vi "MainPanel_20170525.vi"() -> (0 "ErrorOut":errorcluster)   [LabVIEW 2018] (continued)
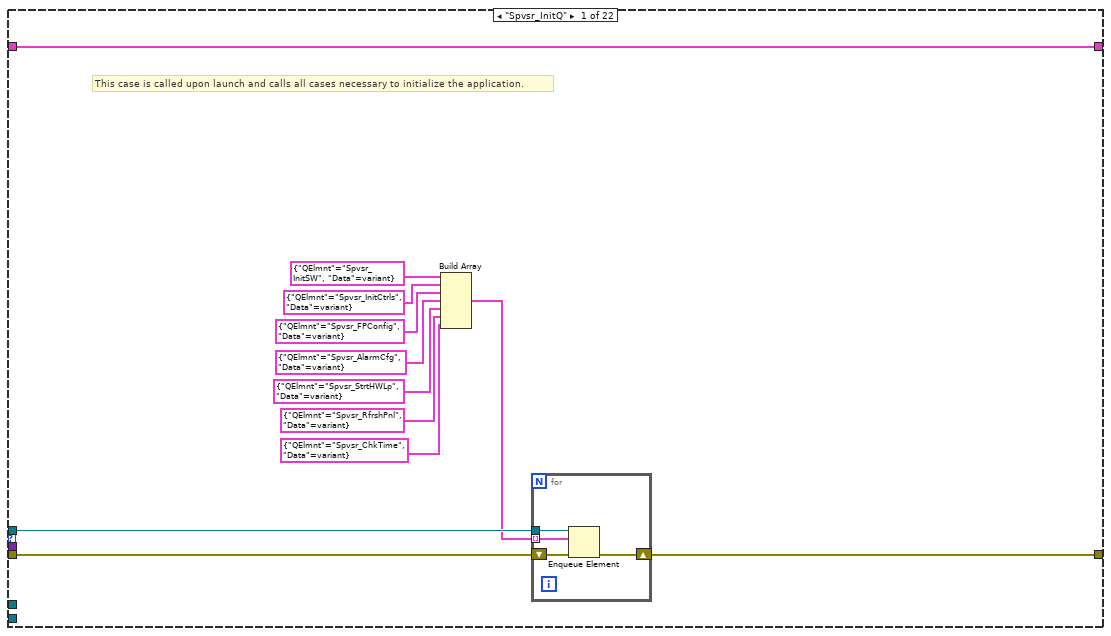
[diagram p3: hidden frame]
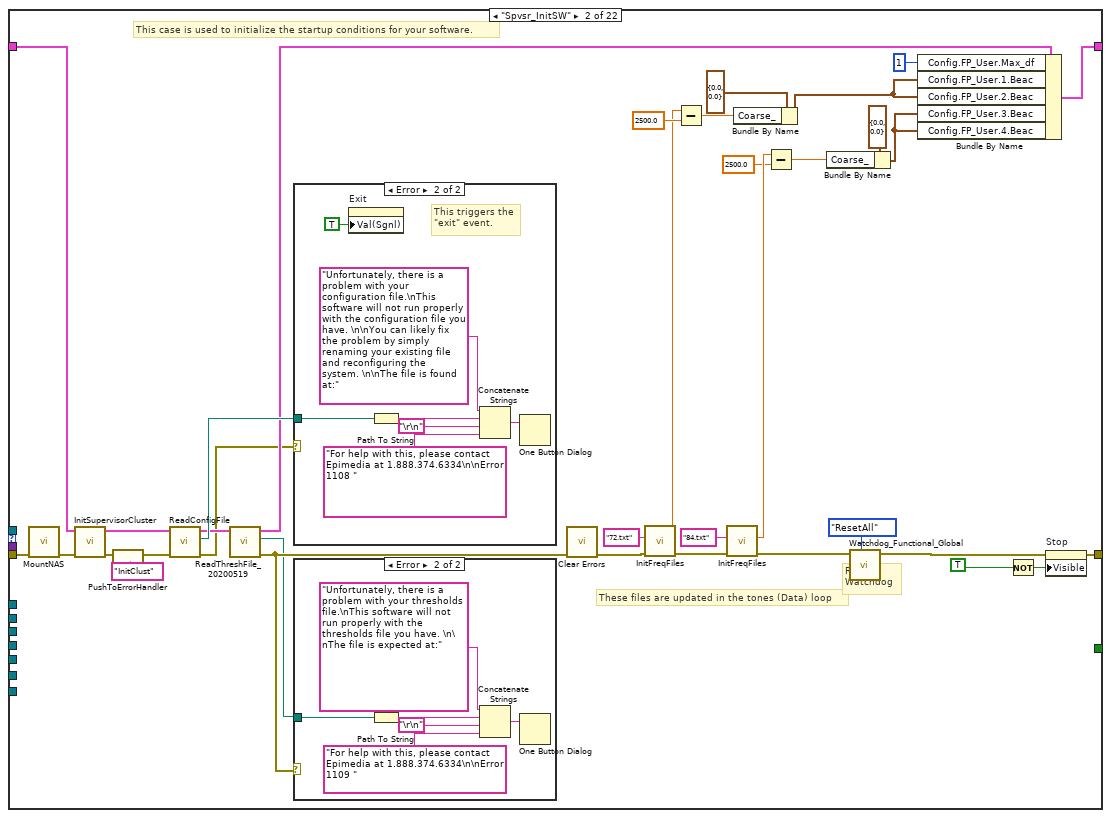
[diagram p4: hidden frame]
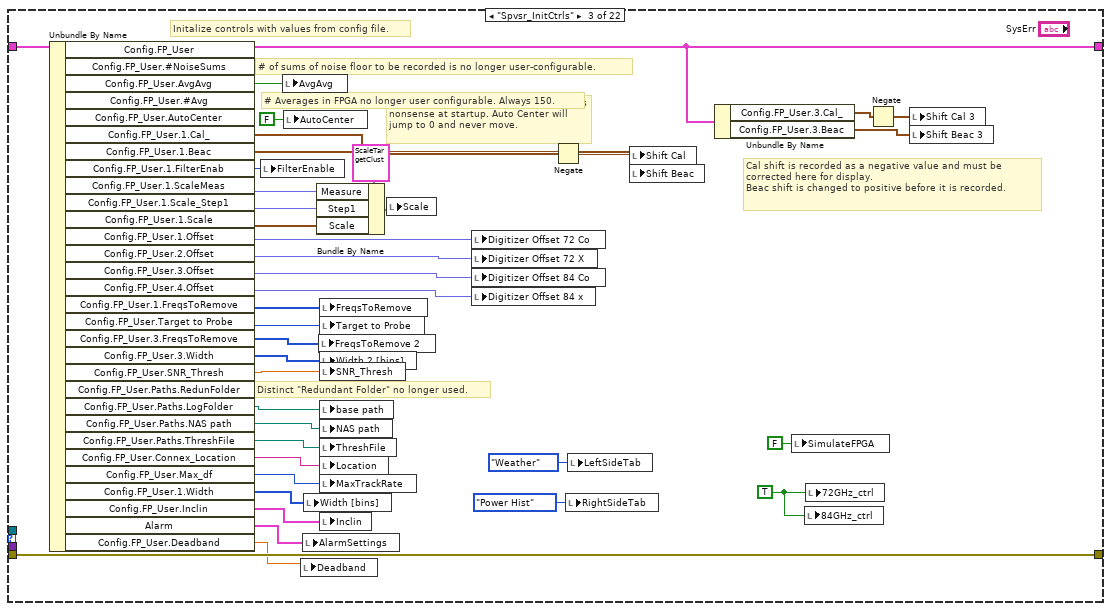
[diagram p7: hidden frame]
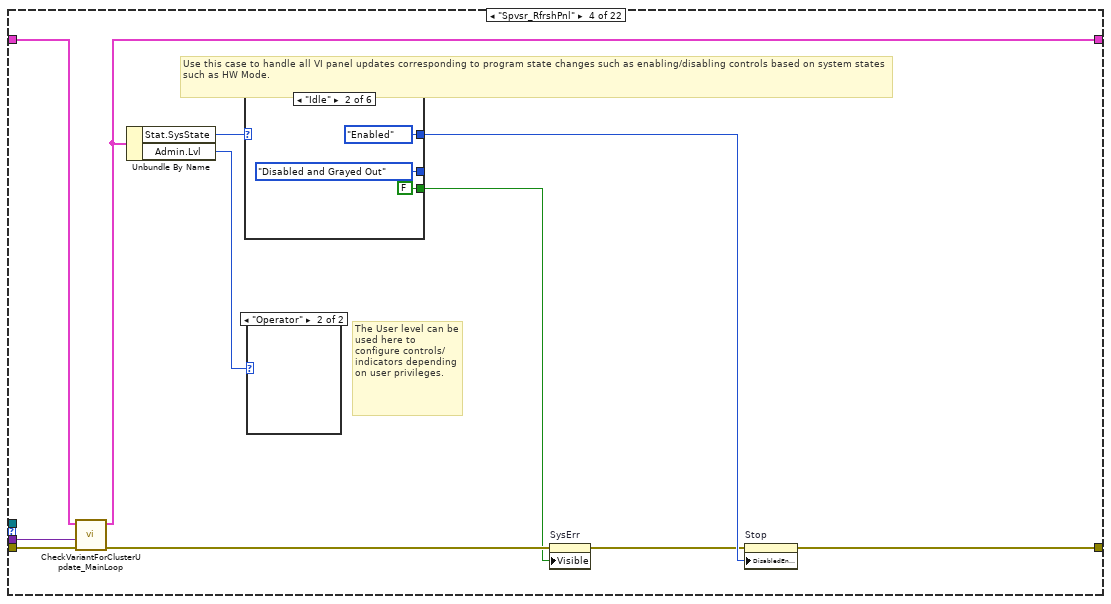
[diagram p8: hidden frame]
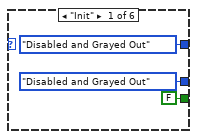
[diagram p10: hidden frame]
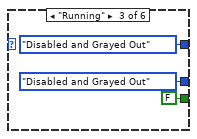
[diagram p11: hidden frame]
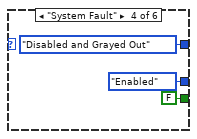
[diagram p12: hidden frame]
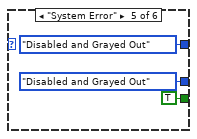
[diagram p13: hidden frame]
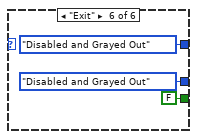
[diagram p14: hidden frame]
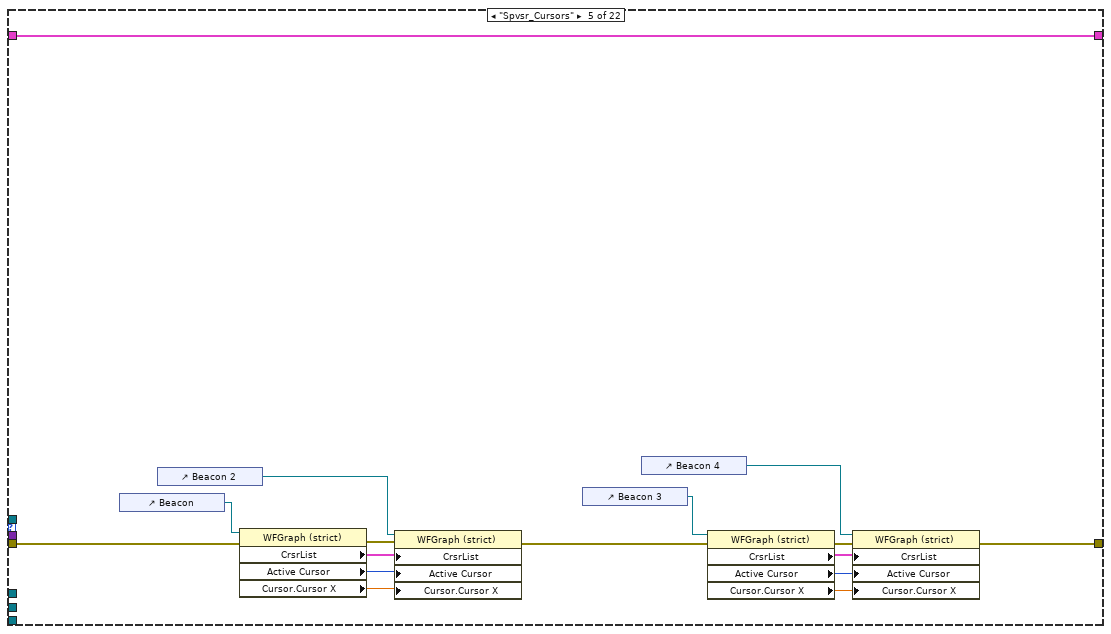
[diagram p15: hidden frame]
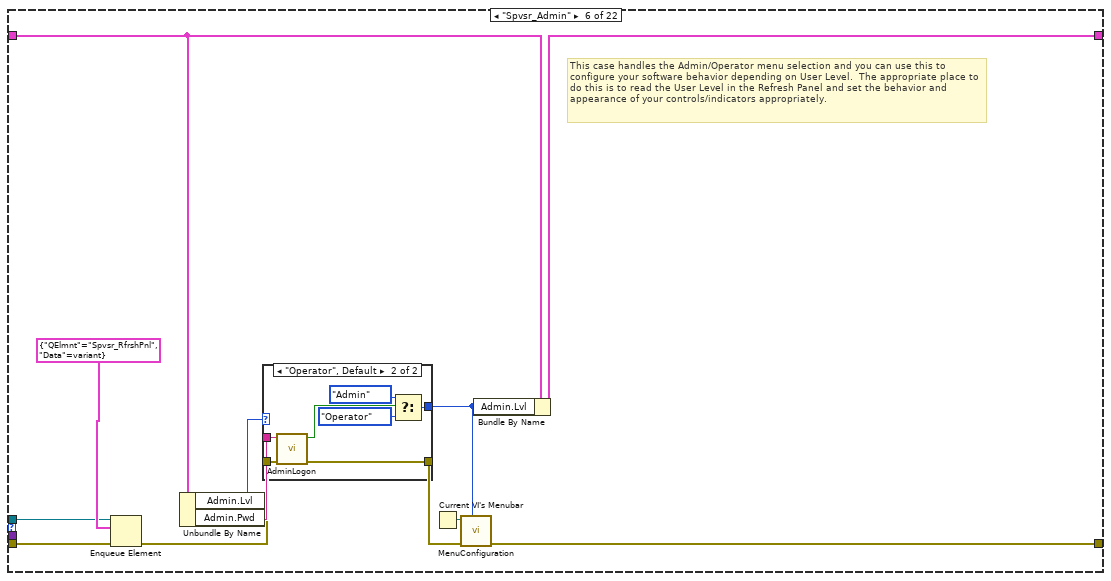
[diagram p16: hidden frame]
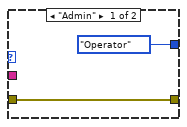
[diagram p17: hidden frame]
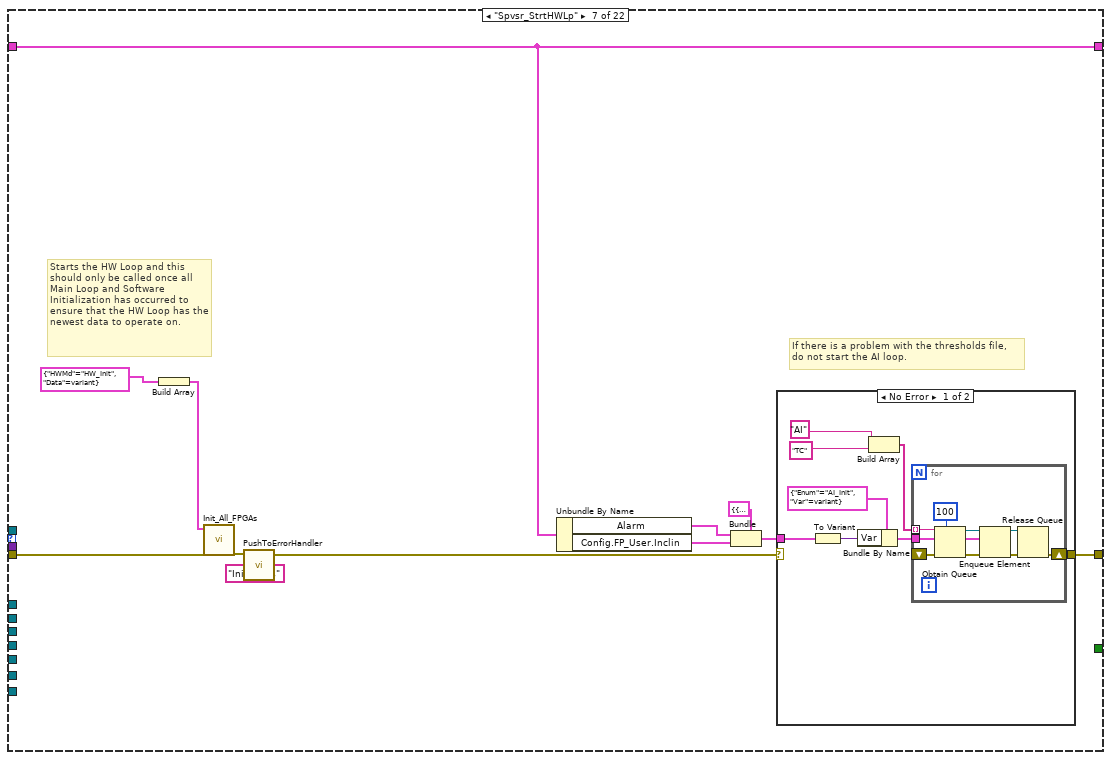
[diagram p18: hidden frame]
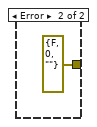
[diagram p19: hidden frame]
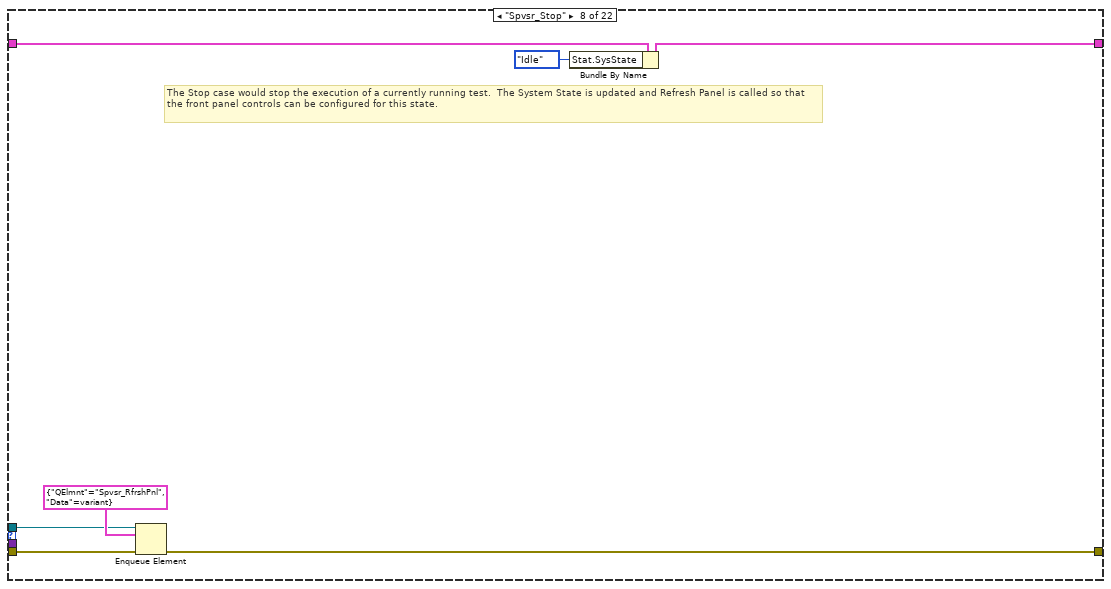
[diagram p20: hidden frame]
        n515 = Variant To Data(error in=w1165, type=T62 {"TCData"={"TimeStamp"=0.0, "TimeString"="", "TC0_LP1_Hi"=0.0, "TC1_LP1_MidHi"=0.0, "TC2_LP1_Mid"=0.0, "TC3_LP1_LoMid"=0.0, "TC4_LP1_Lo"=0.0, "TC5_LP2_Hi"=0.0, "TC6_LP2_MidHi"=0.0, "TC7_LP2_Mid"=0.0, "TC8_LP2_LoMid"=0.0, "TC9_LP2_Lo"=0.0, "TC10_HVAC_Cond_In"=0.0, "TC11_HVAC_Cond_Out"=0.0, "TC12_Gen_Exhaust"=0.0, "TC13_Amb_Inter"=0.0, "TC14_Unused"=0.0, "TC15_Unused"=0.0, "TC16_Unused"=0.0, "TC17_Unused"=0.0, "TC18_Unused"=0.0, "TC19_Unused"=0.0, "TC20_Unused"=0.0, "TC21_Unused"=0.0, "TC22_Unused"=0.0, "TC23_Unused"=0.0, "TC24_Unused"=0.0, "TC25_Unused"=0.0, "TC26_Unused"=0.0, "TC27_Unused"=0.0, "TC28_Unused"=0.0, "TC29_Unused"=0.0, "TC30_Unused"=0.0, "TC31_Unused"=0.0}, "All_TC_ErrorStatus"={"TC 0"={"RX?"=FALSE, "Warn"=FALSE, "Error"=FALSE, "Enabl"=FALSE, "Source"=""}, "TC 1"={"RX?"=FALSE, "Warn"=FALSE, "Error"=FALSE, "Enabl"=FALSE, "Source"=""}, "TC 2"={"RX?"=FALSE, "Warn"=FALSE, "Error"=FALSE, "Enabl"=FALSE, "Source"=""}, "TC 3"={"RX?"=FALSE, "Warn"=FALSE, "Error"=FALSE, "Enabl"=FALSE, "Source"=""}, "TC 4"={"RX?"=FALSE, "Warn"=FALSE, "Error"=FALSE, "Enabl"=FALSE, "Source"=""}, "TC 5"={"RX?"=FALSE, "Warn"=FALSE, "Error"=FALSE, "Enabl"=FALSE, "Source"=""}, "TC 6"={"RX?"=FALSE, "Warn"=FALSE, "Error"=FALSE, "Enabl"=FALSE, "Source"=""}, "TC 7"={"RX?"=FALSE, "Warn"=FALSE, "Error"=FALSE, "Enabl"=FALSE, "Source"=""}, "TC 8"={"RX?"=FALSE, "Warn"=FALSE, "Error"=FALSE, "Enabl"=FALSE, "Source"=""}, "TC 9"={"RX?"=FALSE, "Warn"=FALSE, "Error"=FALSE, "Enabl"=FALSE, "Source"=""}, "TC 10"={"RX?"=FALSE, "Warn"=FALSE, "Error"=FALSE, "Enabl"=FALSE, "Source"=""}, "TC 11"={"RX?"=FALSE, "Warn"=FALSE, "Error"=FALSE, "Enabl"=FALSE, "Source"=""}, "TC 12"={"RX?"=FALSE, "Warn"=FALSE, "Error"=FALSE, "Enabl"=FALSE, "Source"=""}, "TC 13"={"RX?"=FALSE, "Warn"=FALSE, "Error"=FALSE, "Enabl"=FALSE, "Source"=""}, "TC 14"={"RX?"=FALSE, "Warn"=FALSE, "Error"=FALSE, "Enabl"=FALSE, "Source"=""}, "TC 15"={"RX?"=FALSE, "Warn"=FALSE, "Error"=FALSE, "Enabl"=FALSE, "Source"=""}, "TC 16"={"RX?"=FALSE, "Warn"=FALSE, "Error"=FALSE, "Enabl"=FALSE, "Source"=""}, "TC 17"={"RX?"=FALSE, "Warn"=FALSE, "Error"=FALSE, "Enabl"=FALSE, "Source"=""}, "TC 18"={"RX?"=FALSE, "Warn"=FALSE, "Error"=FALSE, "Enabl"=FALSE, "Source"=""}, "TC 19"={"RX?"=FALSE, "Warn"=FALSE, "Error"=FALSE, "Enabl"=FALSE, "Source"=""}, "TC 20"={"RX?"=FALSE, "Warn"=FALSE, "Error"=FALSE, "Enabl"=FALSE, "Source"=""}}}, Variant=w1164) -> (data=w1162:T62, error out=w1159:errorcluster)
        n516 = Unbundle By Name(w1162) -> ("TCData"=w1161:T63)  [unwired: 1 out]
        n517 = call "SortTC_Display.vi"("TCData"=w1161) -> ("TCsDisplay"=w1158:T70)  [unwired: 10 in]
        n518 = Unbundle By Name(w1158) -> ("TC13_Tamb_Interior"=→"ConnextIntTemp":dbl, "TC12_Gen_Exhaust"=→"GeneratorExhaust":dbl)
      }
      frame "FP_PWR_Hist" {
        n519 = Unbundle By Name(w1179) -> ("PwrHist.72Co"=w1178:T68, "PwrHist.72X"=w1177:T68, "PwrHist.84Co"=w1176:T68, "PwrHist.84X"=w1175:T68)
        n520 = Unbundle By Name(w1178) -> ("Cal Smooth"=w1174:dbl, "Beac Smooth"=w1173:dbl)
        n521 = Unbundle By Name(w1177) -> ("Cal Smooth"=w1172:dbl, "Beac Smooth"=w1171:dbl)
        n522 = Unbundle By Name(w1176) -> ("Cal Smooth"=w1170:dbl, "Beac Smooth"=w1169:dbl)
        n523 = Unbundle By Name(w1175) -> ("Cal Smooth"=w1168:dbl, "Beac Smooth"=w1167:dbl)
        n524 = Bundle("Cal Smooth"=w1174, "Beac Smooth"=w1173, "Cal Smooth"=w1172, "Beac Smooth"=w1171, "Cal Smooth"=w1170, "Beac Smooth"=w1169, "Cal Smooth"=w1168, "Beac Smooth"=w1167) -> (→"Combined Power History":T6)  [unwired: 1 in]
      }
      frame "FP_Alarm" {
        w1214 = refnum<vi> refnum ("element")
        # "0: TC13\n1-8: AI1-6,18-19\n9-11: TE1-TE3\n12-15: ADAM1-ADAM4\n\n16: 72Co BeacFreq\n17: Placeholder\n18: 84 Co BeacFreq\n19: Placeholder\n \n20: 72Co CalFreq\n21: Placeholder\n22: 84Co CalFreq\n23: Placeholder\n \n24: 72Co CalTonePwr\n25: 72X CalTonePwr\n26: 84Co CalTonePwr\n27: 84X CalTonePwr\n\n28: SNR Timer"
        # "From Log Loop"
        n525 = Variant To Data(error in=w1252, type=T65 {"Alarms"={"Green"=TRUE, "Rx_Yell"=FALSE, "Cx_Yell"=FALSE, "Red"=FALSE, "Source"=""}, "SerialMeas"={"TE_Air"=0.0, "TE_Bottom"=0.0, "TE_Front"=0.0, "ADAM-Co"=0.0, "ADAM-XPol"=0.0, "ADAM-CalEncl"=0.0, "ADAM-Noise"=0.0}, "AllAlarms"=[], "Elapsed_SNR_Timer"=0.0, "Saturation"={"84"=[], "72"=[]}}, Variant=w1251) -> (data=w1250:T65, error out=w1201:errorcluster)
        n526 = Unbundle By Name(w1250) -> ("Alarms"=w1182:T21, "Elapsed_SNR_Timer"=→"Elapsed_SNR_Timer":dbl, "AllAlarms"=w1241:T61[], "SerialMeas"=w1249:T66, "Saturation"=w1187:T67)
        n527 = control-ref of="MeasMax"() -> (w1208:refnum<vi>)
        n528 = control-ref of="1_Max"() -> (w1207:refnum<vi>)
        n529 = control-ref of="4_Max"() -> (w1206:refnum<vi>)
        n530 = control-ref of="5_Max"() -> (w1205:refnum<vi>)
        n531 = control-ref of="6_Max"() -> (w1204:refnum<vi>)
        n532 = control-ref of="7_Max"() -> (w1203:refnum<vi>)
        n533 = Unbundle By Name(w1249) -> ("TE_Air"=→"TE_Air":dbl, "TE_Bottom"=→"TE_Bottom":dbl, "TE_Front"=→"TE_Front":dbl, "ADAM-Co"=→"ADAM-Co":dbl, "ADAM-XPol"=→"ADAM-XPol":dbl, "ADAM-CalEncl"=→"ADAM-CalEncl":dbl, "ADAM-Noise"=→"ADAM-Noise":dbl)
        n534 = Unbundle By Name(w1187) -> ("84"=w1199:bool[])
        n535 = Build Array(w1208, w1207, w1206, w1205, w1204, w1203) -> (w1202:refnum<vi>[])
        n536 = call "Saturation_Indicator_Color_Code.vi"("SaturationStatus"=w1199, "IndicatorRefs"=w1202) -> ("Error"=w1190:errorcluster)  [unwired: 9 in]
        n537 = Unbundle By Name(w1182) -> ("Green"=→"Green":bool, "Rx_Yell"=→"Rx_Yell":bool, "Cx_Yell"=→"Cx_Yell":bool, "Red"=→"Red":bool)
        n538 = control-ref of="MeasMax"() -> (w1191:refnum<vi>)
        n539 = control-ref of="1_Max"() -> (w1192:refnum<vi>)
        n540 = control-ref of="4_Max"() -> (w1193:refnum<vi>)
        n541 = control-ref of="5_Max"() -> (w1194:refnum<vi>)
        n542 = control-ref of="6_Max"() -> (w1195:refnum<vi>)
        n543 = control-ref of="7_Max"() -> (w1196:refnum<vi>)
        n544 = Unbundle By Name(w1187) -> ("72"=w1198:bool[])
        n545 = Build Array(w1191, w1192, w1193, w1194, w1195, w1196) -> (w1197:refnum<vi>[])
        n546 = control-ref of="ConnextIntTemp"() -> (w1230:refnum<vi>)
        n547 = control-ref of="-5V"() -> (w1231:refnum<vi>)
        n548 = control-ref of="+5"() -> (w1232:refnum<vi>)
        n549 = control-ref of="+6"() -> (w1233:refnum<vi>)
        n550 = control-ref of="+12"() -> (w1234:refnum<vi>)
        n551 = control-ref of="+15"() -> (w1235:refnum<vi>)
        n552 = control-ref of="+28"() -> (w1236:refnum<vi>)
        n553 = control-ref of="InclAz"() -> (w1237:refnum<vi>)
        n554 = control-ref of="InclEl"() -> (w1238:refnum<vi>)
        n555 = control-ref of="TE_Air"() -> (w1239:refnum<vi>)
        n556 = control-ref of="TE_Bottom"() -> (w1228:refnum<vi>)
        n557 = control-ref of="TE_Front"() -> (w1221:refnum<vi>)
        n558 = call "Saturation_Indicator_Color_Code.vi"("SaturationStatus"=w1198, "IndicatorRefs"=w1197) -> ("Error"=w1189:errorcluster)  [unwired: 9 in]
        n559 = Merge Errors(w1190, w1189) -> (w1188:errorcluster)
        n560 = Build Array(w1230, w1231, w1232, w1233, w1234, w1235, w1236, w1237, w1238, w1239, w1228, w1221) -> (w1224:refnum<vi>[])
        n561 = control-ref of="ADAM-Co"() -> (w1229:refnum<vi>)
        n562 = control-ref of="ADAM-XPol"() -> (w1227:refnum<vi>)
        n563 = control-ref of="ADAM-CalEncl"() -> (w1226:refnum<vi>)
        n564 = control-ref of="ADAM-Noise"() -> (w1225:refnum<vi>)
        n565 = control-ref of="72CoBeacFrq"() -> (w1220:refnum<vi>)
        n566 = control-ref of="84CoBeacFrq"() -> (w1217:refnum<vi>)
        n567 = control-ref of="72CoCalFrq"() -> (w1216:refnum<vi>)
        n568 = control-ref of="84CoCalFrq"() -> (w1215:refnum<vi>)
        n569 = control-ref of="MaxValue_Cal_72Co"() -> (w1213:refnum<vi>)
        n570 = control-ref of="MaxValue_Cal_72X"() -> (w1212:refnum<vi>)
        n571 = control-ref of="MaxValue_Cal_84Co"() -> (w1211:refnum<vi>)
        n572 = control-ref of="MaxValue_Cal_84X"() -> (w1210:refnum<vi>)
        n573 = control-ref of="Elapsed_SNR_Timer"() -> (w1218:refnum<vi>)
        n574 = Build Array(w1229, w1227, w1226, w1225, w1220, w1214, w1217, w1214, w1216, w1214, w1215, w1214, w1213, w1212, w1211, w1210, w1218) -> (w1223:refnum<vi>[])
        n575 = Build Array (concatenate)(w1224, w1223) -> (w1222:refnum<vi>[])
        n576 = Merge Errors(w1188, w1201) -> (w1200:errorcluster)
        n577 = for {
          tunnel: w1222 -> [w1261] mode=indexing
          tunnel: w1241 -> [w1257] mode=indexing
          shift-right: [w1254] -> w1240
          shift-left: w1200 -> [w1253]
          n578 = To More Specific Class(target class=refnum<vi> refnum ("AI0_Inclinometer"), reference=w1261) -> (specific class reference=w1260:refnum<vi>, error out=w1255:errorcluster)  [unwired: 1 in]
          n579 = call "Indicator_Error_Color.vi"("AI 0"=w1257) -> ("Label.Text Colors:BG Color"=w1258:u32)  [unwired: 10 in]
          n580 = property on="Property Node" class="DigNum"(reference=w1260, error in=w1255, "NumText.BGColor"=w1258) -> (error out=w1256:errorcluster)  [unwired: 1 out]
          n581 = Merge Errors(w1253, w1256) -> (w1254:errorcluster)
        }
      }
      frame "FP_Exit" {
        n582 = Release Queue(queue=w1265, error in (no error)=w1264) -> (error out=w1263:errorcluster)  [unwired: 1 in, 2 out]
      }
    }
    "FP_Count" <- w900
  }
  n583 = disable-structure shown="Enabled" {
    disable-tunnel: w135 -> [w1272 w1273]
    disable-tunnel: w65 -> [w1271 _]
    disable-tunnel: [w1270 w1273] -> w127
    disable-tunnel: w118 -> [w1269 _]
    disable-tunnel: TargetNumber."2" ("FPGA.Target") -> [w1268 _]
    disable-tunnel: w75 -> [w1267 _]
    frame Enabled {
      n584 = call "HW_Loop_20181101.vi"("ErrorLocation"=w1269, "error in (no error)"=w1272, "10MHzPLL?"=w1267, "FPGA.Target"=w1268, "Queue in"=w1271) -> ("error out"=w1270:errorcluster)  [unwired: 6 in]
    }
    frame Disabled {
    }
  }
  n585 = call "HW_Loop_20181101.vi"("ErrorLocation"=w119, "error in (no error)"=w153, "10MHzPLL?"=w75, "FPGA.Target"=TargetNumber."1", "Queue in"=w154) -> ("error out"=w152:errorcluster)  [unwired: 6 in]
  n586 = property class="VI"(error in=w53) -> (error out=w60:errorcluster, "Panel"=w58:refnum<vi>)  [unwired: 1 in, 1 out]
  n587 = property class="VI"(error in=w17) -> (error out=w25:errorcluster, "Panel"=w27:refnum<vi>)  [unwired: 1 in, 1 out]
  n588 = property class="VI"(error in=w43) -> (error out=w50:errorcluster, "Panel"=w52:refnum<vi>)  [unwired: 1 in, 1 out]
  n589 = property class="VI"(error in=w29) -> (error out=w37:errorcluster, "Panel"=w39:refnum<vi>)  [unwired: 1 in, 1 out]
  n590 = property class="Pnl"(reference=w58, error in=w60) -> (reference out=w59:refnum<vi>, error out=w61:errorcluster, "Panes[]"=w64:refnum<vi>[])
  n591 = property class="Pnl"(reference=w27, error in=w25) -> (reference out=w26:refnum<vi>, error out=w24:errorcluster, "Panes[]"=w21:refnum<vi>[])
  n592 = property class="Pnl"(reference=w52, error in=w50) -> (reference out=w51:refnum<vi>, error out=w49:errorcluster, "Panes[]"=w46:refnum<vi>[])
  n593 = property class="Pnl"(reference=w39, error in=w37) -> (reference out=w38:refnum<vi>, error out=w36:errorcluster, "Panes[]"=w33:refnum<vi>[])
  n594 = Close Reference(reference=w59, error in (no error)=w61) -> (error out=w62:errorcluster)
  n595 = Close Reference(reference=w26, error in (no error)=w24) -> (error out=w23:errorcluster)
  n596 = Close Reference(reference=w51, error in (no error)=w49) -> (error out=w48:errorcluster)
  n597 = Close Reference(reference=w38, error in (no error)=w36) -> (error out=w35:errorcluster)
  n598 = for {
    tunnel: w64 -> [w1277] mode=indexing
    tunnel: w62 -> [w1276]
    shift-right: [w1275] -> w63
    shift-left: _ -> [_]
    w1274 = T71."Off While Running" ("Horizontal Scrollbar Visibility")
    n599 = property class="Pane"(reference=w1277, error in=w1276, "HorizScrollbarVisibility"=w1274, "VertScrollbarVisibility"=w1274) -> (error out=w1275:errorcluster)  [unwired: 1 out]
  }
  n600 = for {
    tunnel: w21 -> [w1281] mode=indexing
    tunnel: w23 -> [w1280]
    shift-right: [w1279] -> w22
    shift-left: _ -> [_]
    w1278 = T71."Off While Running" ("Horizontal Scrollbar Visibility")
    n601 = property class="Pane"(reference=w1281, error in=w1280, "HorizScrollbarVisibility"=w1278, "VertScrollbarVisibility"=w1278) -> (error out=w1279:errorcluster)  [unwired: 1 out]
  }
  n602 = for {
    tunnel: w46 -> [w1285] mode=indexing
    tunnel: w48 -> [w1284]
    shift-right: [w1283] -> w47
    shift-left: _ -> [_]
    w1282 = T71."Off While Running" ("Horizontal Scrollbar Visibility")
    n603 = property class="Pane"(reference=w1285, error in=w1284, "HorizScrollbarVisibility"=w1282, "VertScrollbarVisibility"=w1282) -> (error out=w1283:errorcluster)  [unwired: 1 out]
  }
  n604 = for {
    tunnel: w33 -> [w1289] mode=indexing
    tunnel: w35 -> [w1288]
    shift-right: [w1287] -> w34
    shift-left: _ -> [_]
    w1286 = T71."Off While Running" ("Horizontal Scrollbar Visibility")
    n605 = property class="Pane"(reference=w1289, error in=w1288, "HorizScrollbarVisibility"=w1286, "VertScrollbarVisibility"=w1286) -> (error out=w1287:errorcluster)  [unwired: 1 out]
  }
  n606 = Close Reference(reference=w64, error in (no error)=w63) -> (error out=w107:errorcluster)
  n607 = Close Reference(reference=w21, error in (no error)=w22) -> (error out=w103:errorcluster)
  n608 = Close Reference(reference=w46, error in (no error)=w47) -> (error out=w111:errorcluster)
  n609 = Close Reference(reference=w33, error in (no error)=w34) -> (error out=w105:errorcluster)
  n610 = Build Array(w74, w73, w72) -> (w69:refnum<vi>[])
  n611 = Merge Errors(w159, w158, w152, w127, w150, w137, w147, w120, w109, w3, w66, w121, w112, w117, w110, w111, w107, w105, w103, w106) -> (w71:errorcluster)
  n612 = call "Abort_NASA_VIs.vi"("error in"=w71, "VI_Refs"=w69) -> ("error out"=w70:errorcluster)  [unwired: 9 in]
  n613 = flat-sequence {
    tunnel: [w1290] -> w144
    tunnel: w70 -> [w1290]
    frame #0 {
      n614 = local write "Exit"(FALSE ("Exit")) -> ()
    }
  }
  n615 = call "ExitLabVIEW.vi"("ErrorIn"=w144) -> ("ErrorOut"=→"ErrorOut":errorcluster)  [unwired: 14 out]
